vi "Timestamps to Seconds.vi"(11 "Timestamps":string[](array[string])) -> (3 "Times":dbl[](array[numeric]))   [LabVIEW 2019]
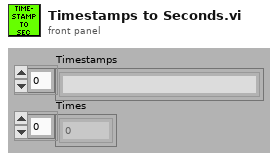
[diagram p1: front panel]
types:
  T1 = cluster{"second":i32, "minute":i32, "hour":i32, "day of month":i32, "month":i32, "year":i32, "day of week":i32, "day of year":i32, "is DST":i32}
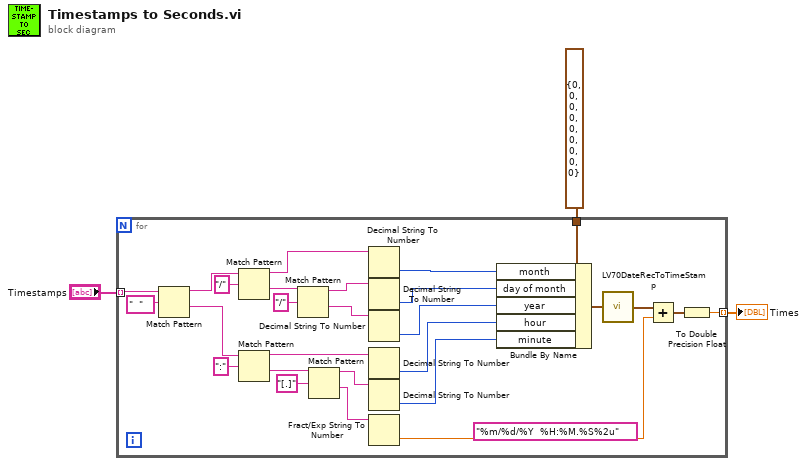
[diagram p0: block diagram]
diagram:
  n1 = for {
    tunnel: "Timestamps" -> [w30] mode=indexing
    tunnel: T1 {"second"=0, "minute"=0, "hour"=0, "day of month"=0, "month"=0, "year"=0, "day of week"=0, "day of year"=0, "is DST"=0} ("date time rec") -> [w28]
    tunnel: [w4] -> w1 mode=indexing
    (unwired) "%m/%d/%Y  %H:%M.%S%2u" ("time format string (%c)")
    n2 = Match Pattern(string=w30, regular expression="  ") -> (before substring=w27:string, after substring=w16:string)  [unwired: 1 in, 2 out]
    n3 = Match Pattern(string=w27, regular expression="/") -> (before substring=w23:string, after substring=w24:string)  [unwired: 1 in, 2 out]
    n4 = Match Pattern(string=w16, regular expression=":") -> (before substring=w13:string, after substring=w14:string)  [unwired: 1 in, 2 out]
    n5 = Match Pattern(string=w24, regular expression="/") -> (before substring=w22:string, after substring=w21:string)  [unwired: 1 in, 2 out]
    n6 = Match Pattern(string=w14, regular expression="[.]") -> (before substring=w12:string, after substring=w7:string)  [unwired: 1 in, 2 out]
    n7 = Decimal String To Number(string=w23) -> (number=w20:i32)  [unwired: 2 in, 1 out]
    n8 = Decimal String To Number(string=w22) -> (number=w19:i32)  [unwired: 2 in, 1 out]
    n9 = Decimal String To Number(string=w21) -> (number=w18:i32)  [unwired: 2 in, 1 out]
    n10 = Decimal String To Number(string=w13) -> (number=w11:i32)  [unwired: 2 in, 1 out]
    n11 = Decimal String To Number(string=w12) -> (number=w10:i32)  [unwired: 2 in, 1 out]
    n12 = Fract/Exp String To Number(string=w7) -> (number=w6:dbl)  [unwired: 3 in, 1 out]
    n13 = Bundle By Name(cluster=w28, "month"=w20, "day of month"=w19, "year"=w18, "hour"=w11, "minute"=w10) -> (w9:T1)
    n14 = call <vilib>:"LV70DateRecToTimeStamp.vi"("date time rec"=w9) -> ("Time Stamp"=w8:timestamp)
    n15 = Add(x=w8, y=w6) -> (x+y=w5:timestamp)
    n16 = To Double Precision Float(number=w5) -> (double precision float=w4:dbl)
  }
  "Times" <- w1
